vi "serialization tests.vi"() -> ()   [LabVIEW 2013, in "tdms logger tests.lvlib"]
uses:
  tdms logger tests.lvlib
  configuration/TDMS datalogger configuration.lvclass
panel:
  out "channels equal":bool
  out "no error":errorcluster
  out "no error":errorcluster
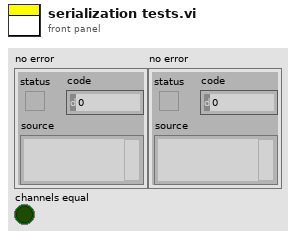
[diagram p1: front panel]
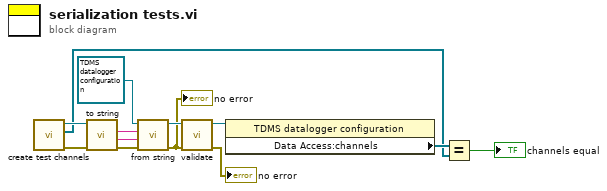
[diagram p0: block diagram]
diagram:
  n1 = call "create test channels.vi"() -> ("error out"=w2:errorcluster, "chans"=w1:refnum<class "TBM channel.lvclass">[], "TDMS datalogger configuration out"=w3:refnum<class "TDMS datalogger configuration.lvclass">)  [unwired: 8 in, 1 out]
  n2 = call-dynamic "to string.vi"("error in"=w2, "TDMS datalogger configuration in"=w3) -> ("error out"=w13:errorcluster, "data"=w12:string, "version"=w11:string)  [unwired: 6 in, 1 out]
  n3 = call-dynamic "from string.vi"("error in"=w13, "data"=w12, "version"=w11, "TDMS datalogger configuration in"=refnum<class "TDMS datalogger configuration.lvclass"> refnum ("TDMS datalogger configuration")) -> ("error out"=w8:errorcluster, "TDMS datalogger configuration out"=w10:refnum<class "TDMS datalogger configuration.lvclass">)  [unwired: 6 in]
  "no error" <- w8
  n4 = call-dynamic "validate.vi"("error in"=w8, "TDMS datalogger configuration in"=w10) -> ("error out"=→"no error":errorcluster, "TDMS datalogger configuration out"=w6:refnum<class "TDMS datalogger configuration.lvclass">)  [unwired: 8 in]
  n5 = property class="TDMS datalogger configuration"(reference=w6) -> ("Data Access:channels"=w5:refnum<class "TBM channel.lvclass">[])  [unwired: 1 in, 2 out]
  n6 = Equal?(x=w5, y=w1) -> (x = y?=→"channels equal":bool)
